vi "xml generate for Q8X.vi"(0 "width1":dbl, 1 "width2":dbl, 2 "single spec":T1={"limit Spec"=array1616x8[12928 elements], "Diff Test Item Name"=["SDD21", "SDD11", "SCD22", "SCC11", "SCD21-SDD21", "NEXT", "ILD_15"], "Spec _Col"=[1, 2, 3, 4, 5, 6, 7]}, 3 "auto get refer point":bool, 4 "input_array_TDD11":string[](array[string]), 5 "input_array_TDD22":string[](array[string]), 6 "input_path_dataSource":path, 7 "input_test_results":bool[](array[boolean]), 8 "show_impspec":string[](array[string]), 10 "路径":path=path "D:/wmgxml.xml", 11 "input_array_time":string[](array[string]), 12 "input_str_label":string, 13 "input_array_impSpec":string[](array[string]), 14 "input_str_CustomerPN":string, 16 "FilePath":string, 17 "FileVer":string, 18 "terminal points":dbl[](array[numeric]), 19 "cable points":dbl[](array[numeric])) -> ()   [LabVIEW 2011]
uses:
  <vilib>/Utility/file.llb/Read From Spreadsheet File (DBL).vi
panel:
  in  "width1 2":dbl
  in  "width2 2":dbl
  in  "cable points 2":dbl[](array[numeric])
  in  "terminal points 4":dbl[](array[numeric])
  in  "auto get refer point 2":bool
  out "terminal points 3":dbl[](array[numeric])
  out "terminal points 2":dbl[](array[numeric])
  out "TestResult":string
  out "TDD":string
  out "NEXT":string
  out "SCC11":string
  out "SCD21-SDD21":string
  out "ILD":string
  out "SDD11":string
  out "SDD21":string
  out "midVar_time":string[](array[string])
  in  "midVar_state":string
  in  "input_str_product":string
  out "midVar_Content":string
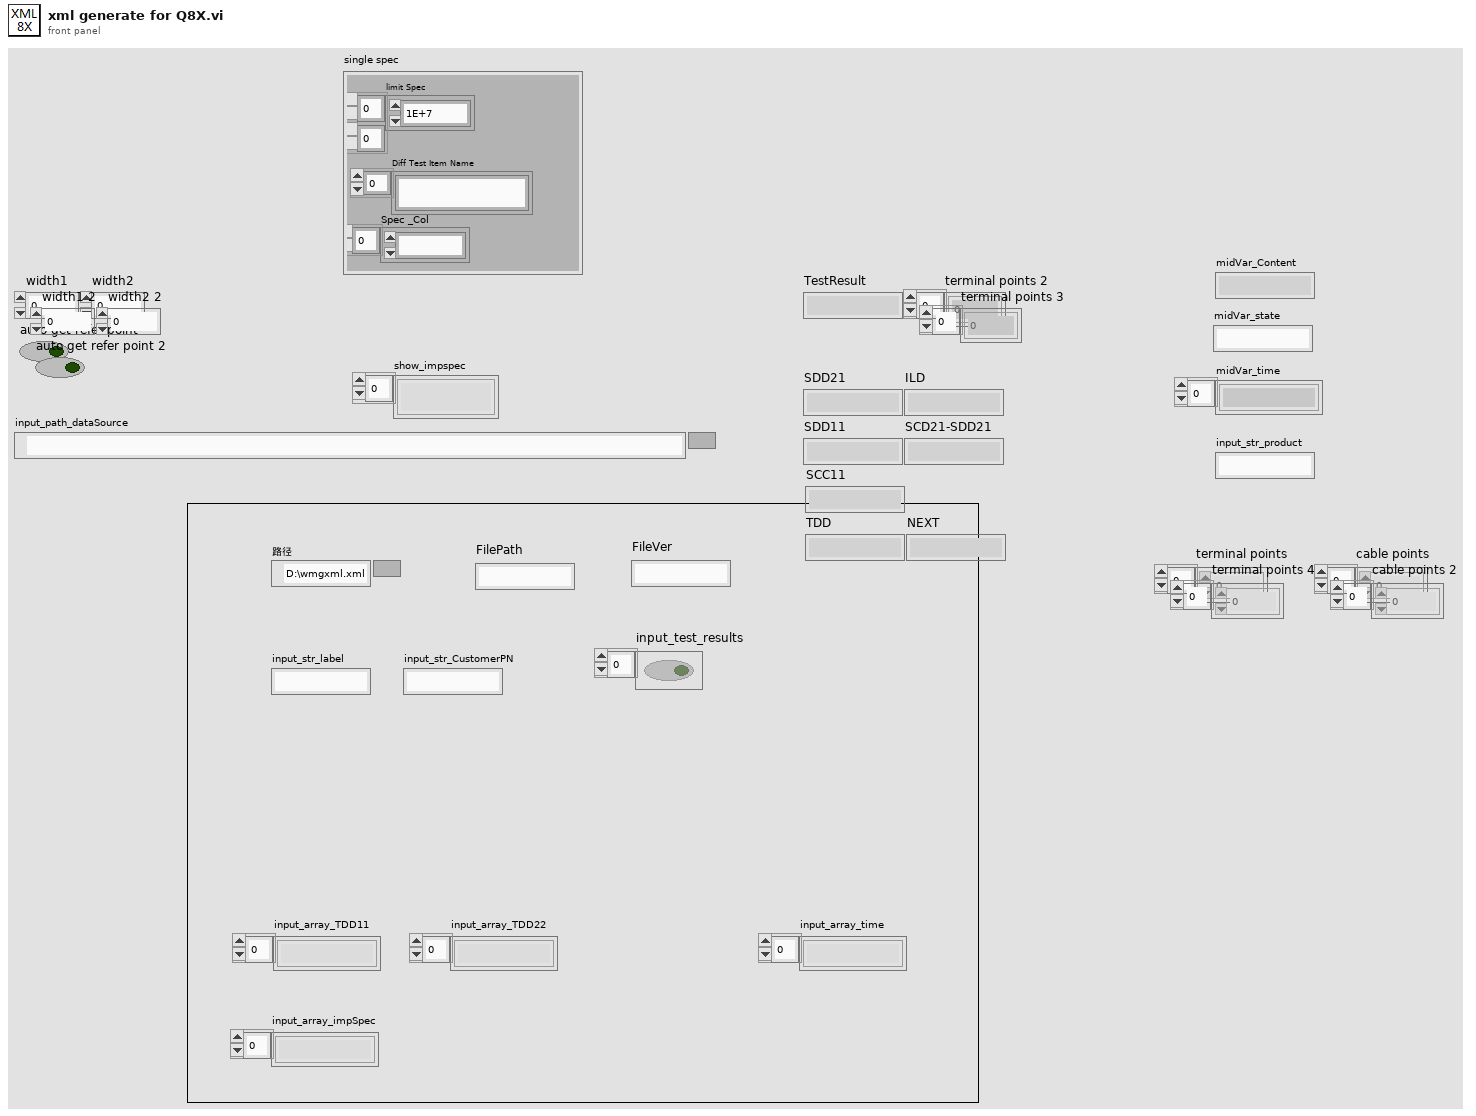
[diagram p1: front panel]
types:
  T1 = cluster{"limit Spec":dbl[][], "Diff Test Item Name":string[], "Spec _Col":i32[]}
  T2 = enum16{"open", "replace", "create", "open or create", "replace or create", "replace or create with confirmation"}
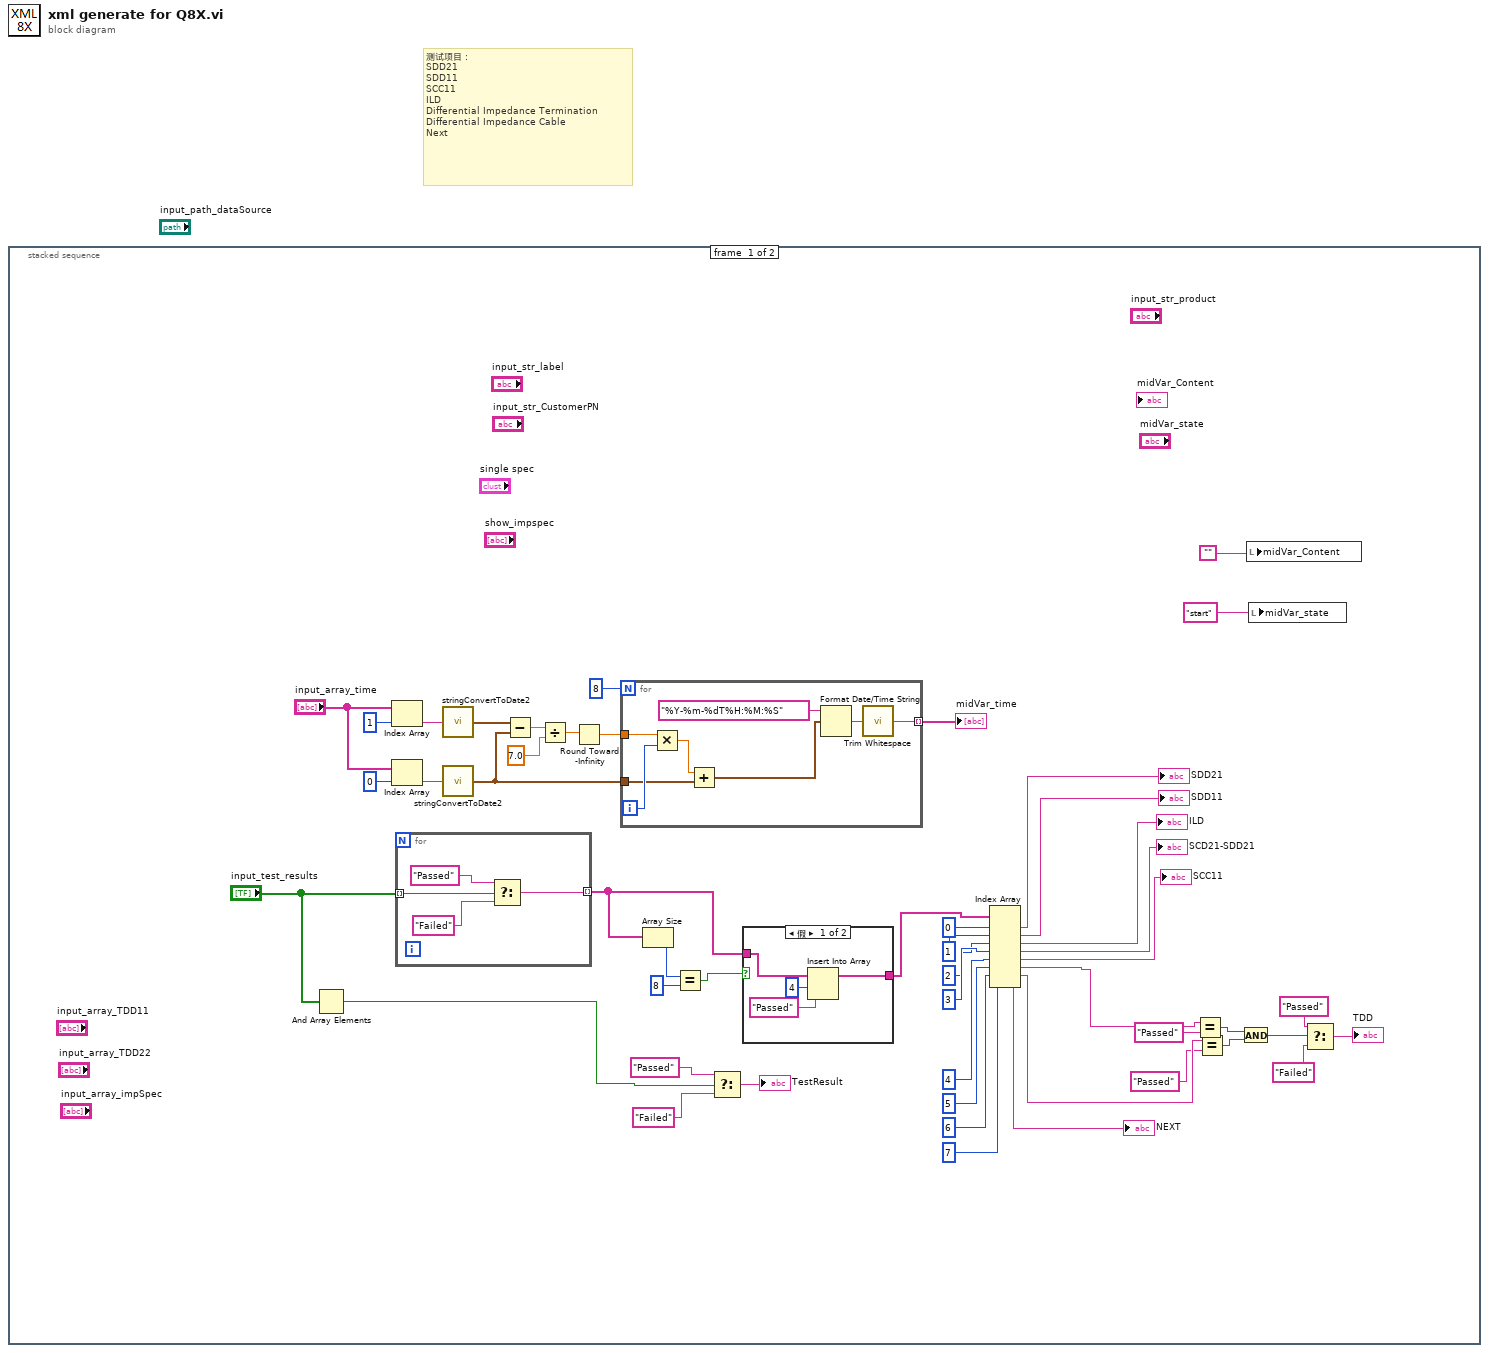
[diagram p0: block diagram]
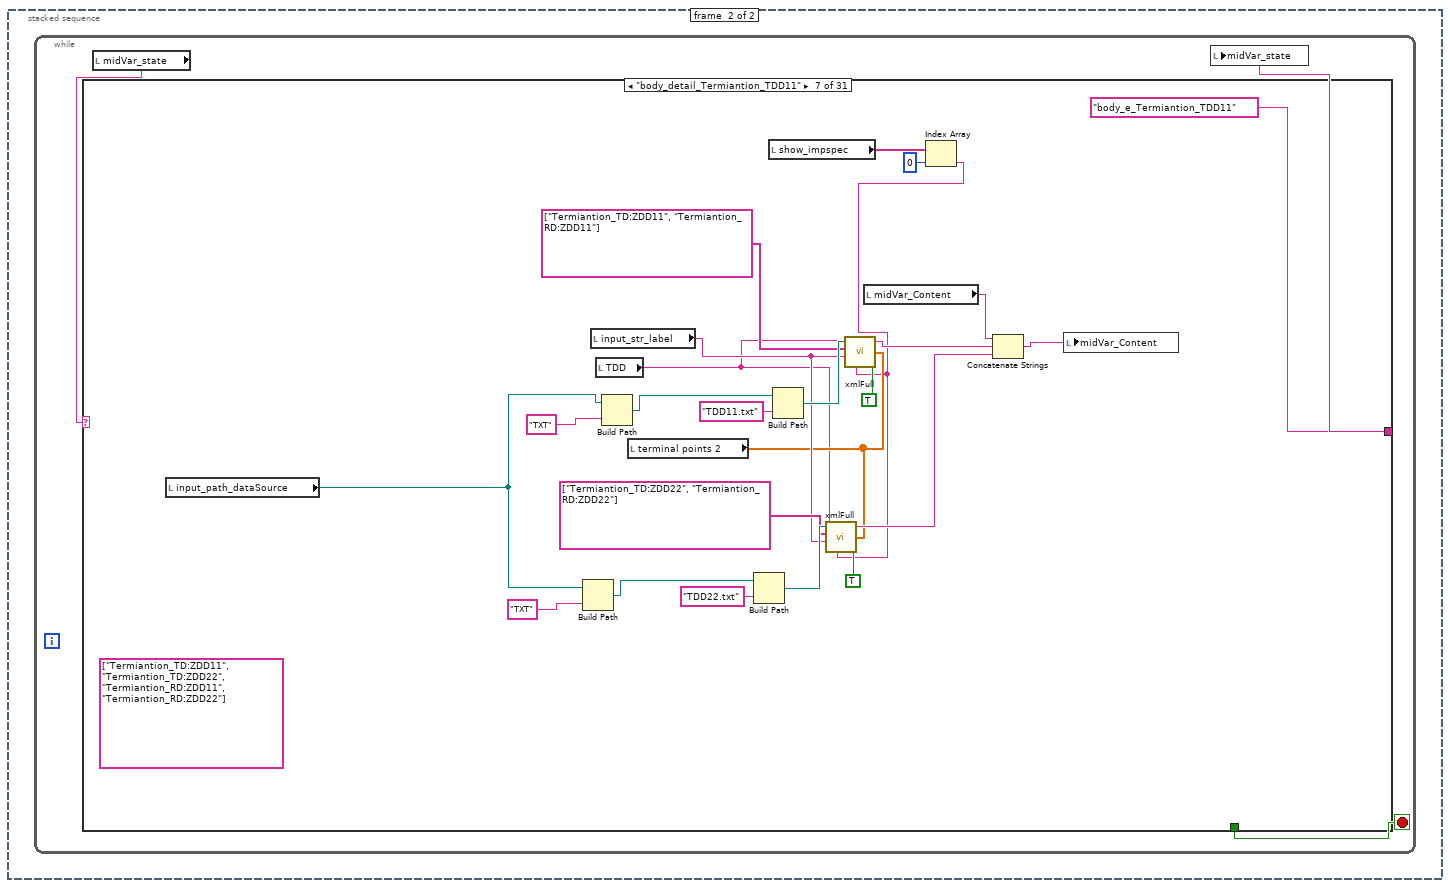
[diagram p3: hidden frame]
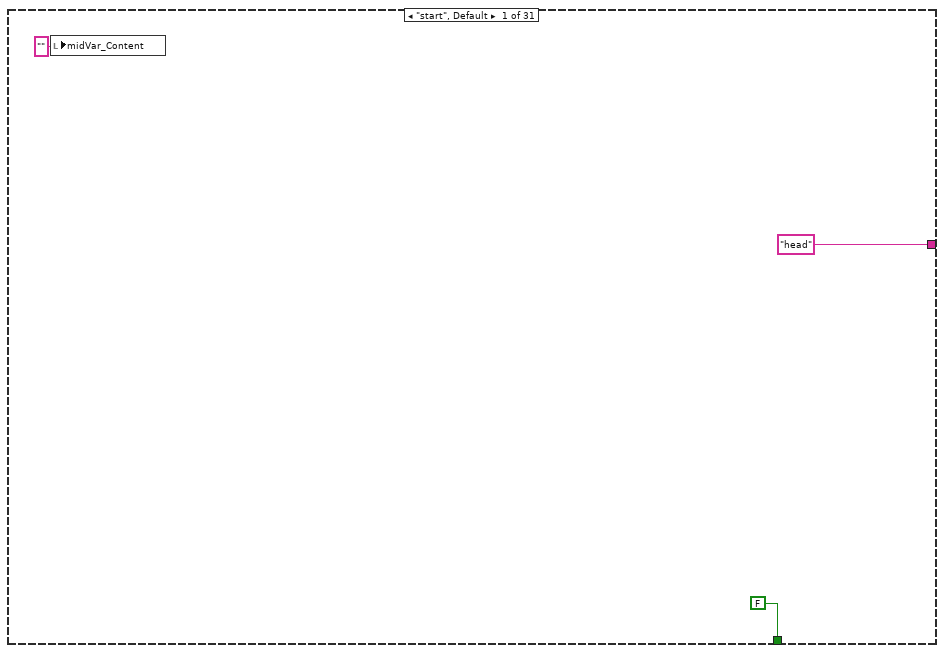
[diagram p4: hidden frame]
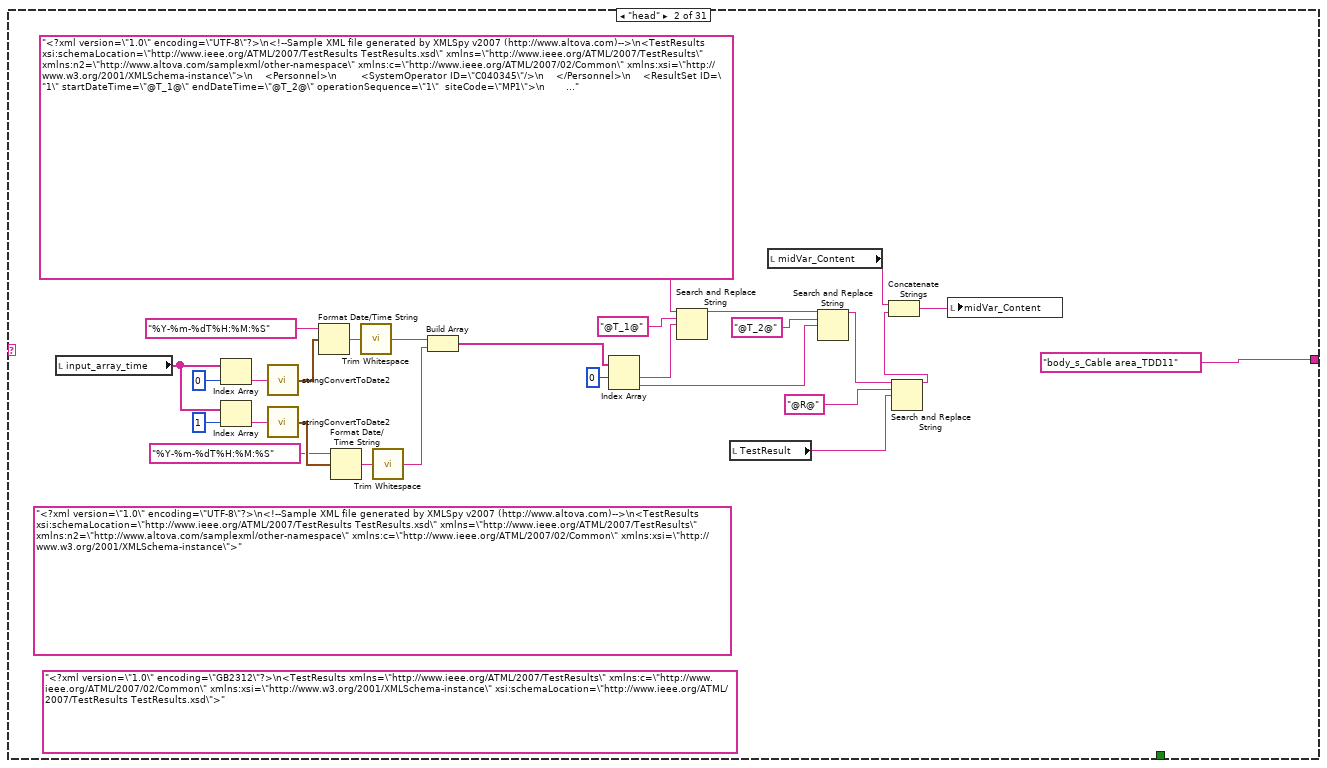
[diagram p5: hidden frame]
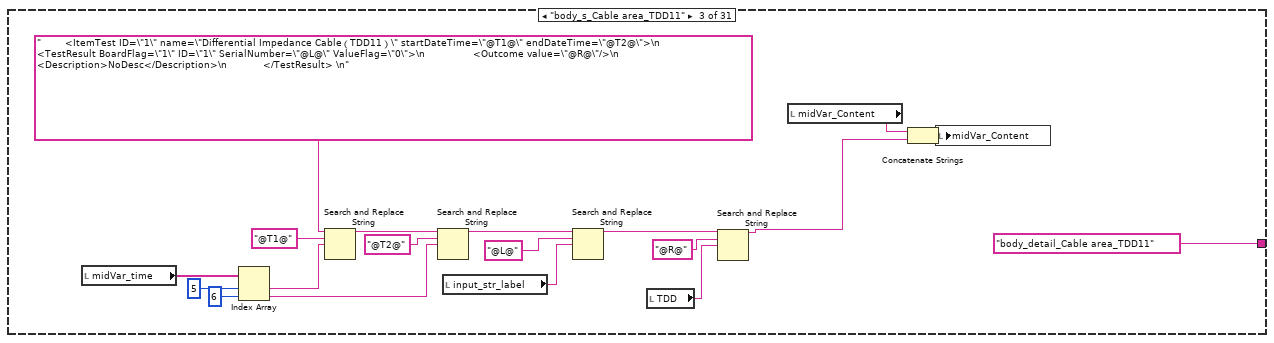
[diagram p6: hidden frame]
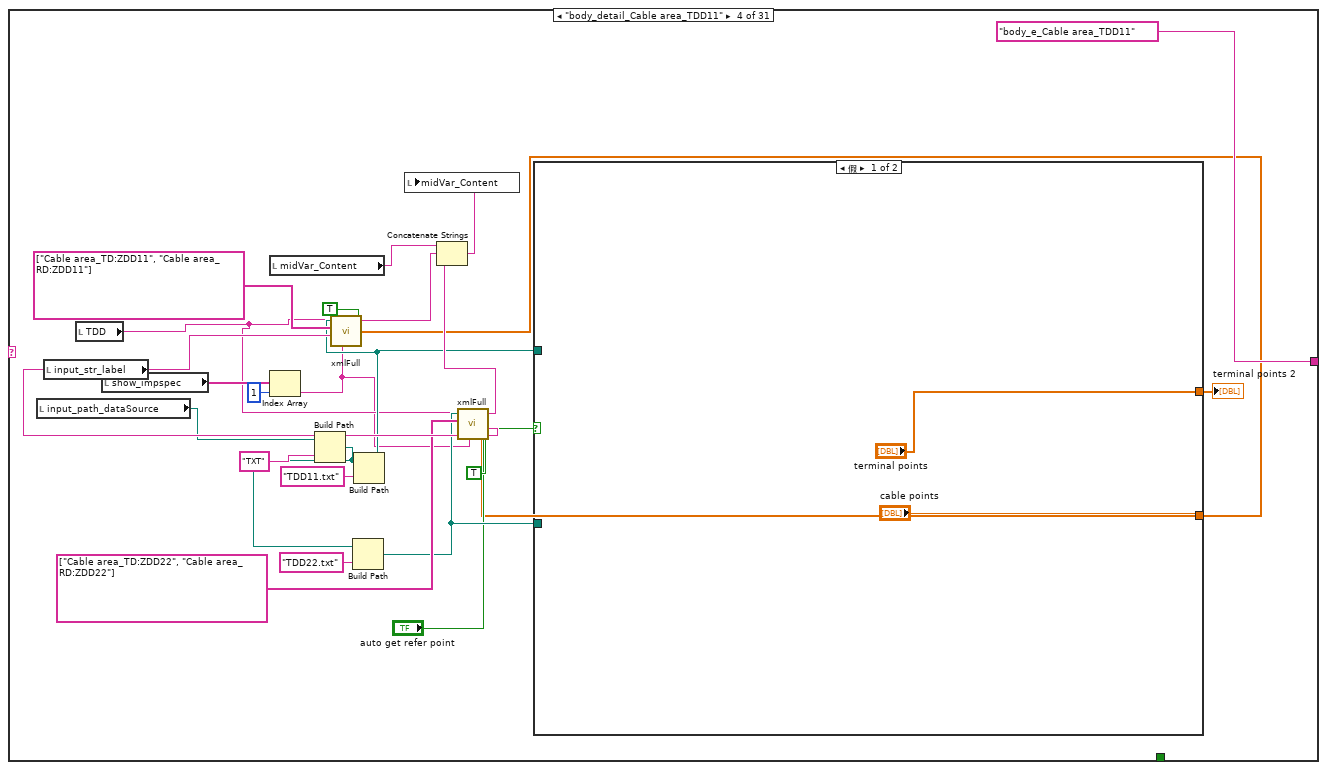
[diagram p7: hidden frame]
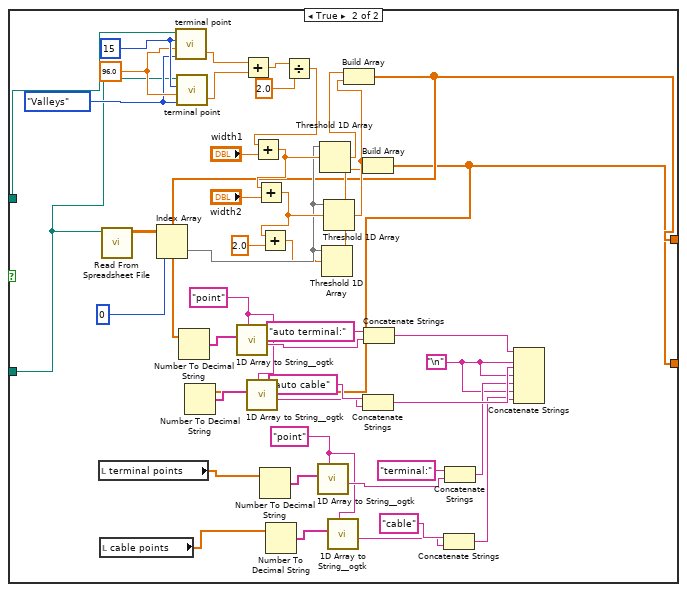
[diagram p8: hidden frame]
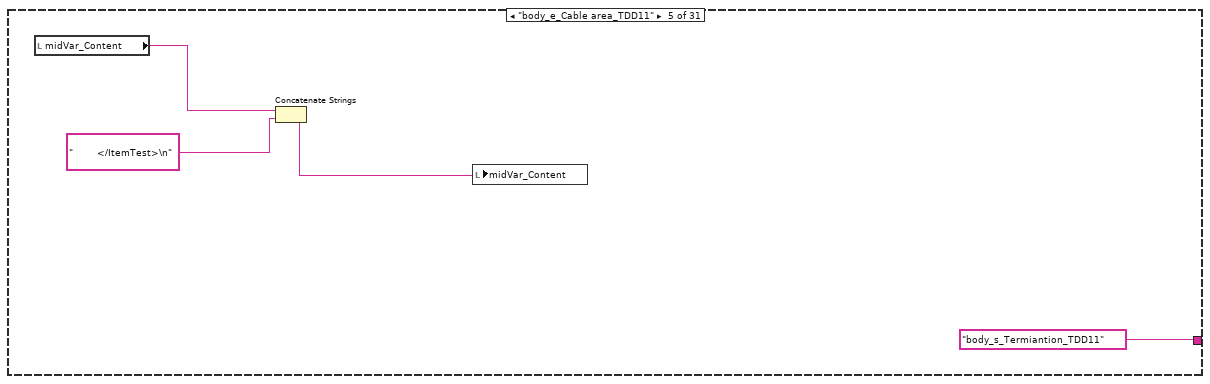
[diagram p9: hidden frame]
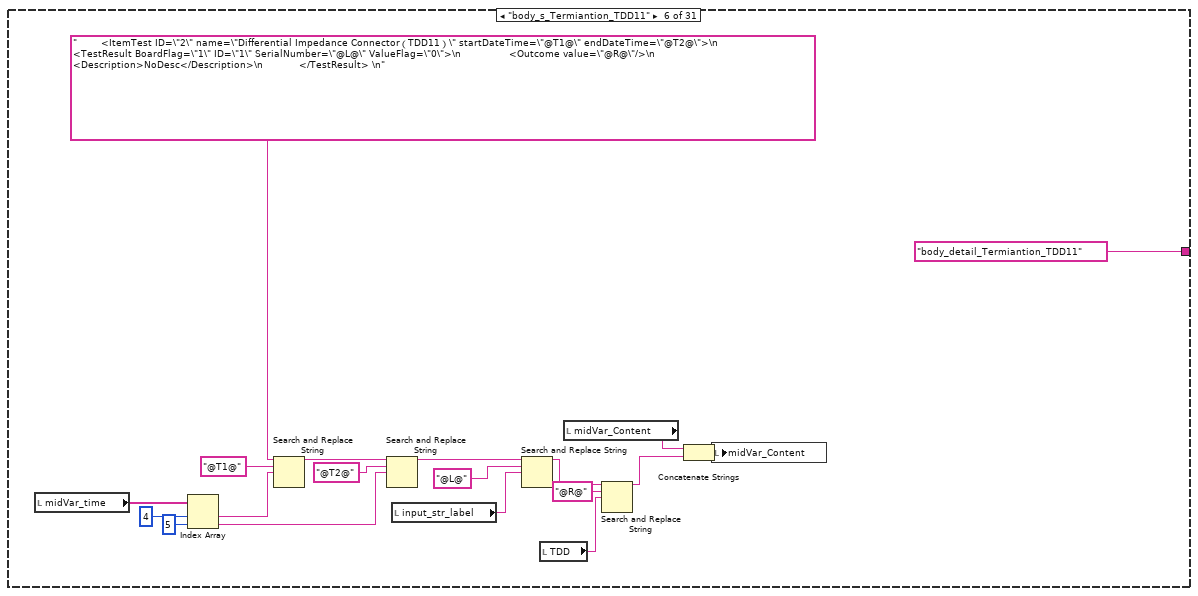
[diagram p10: hidden frame]
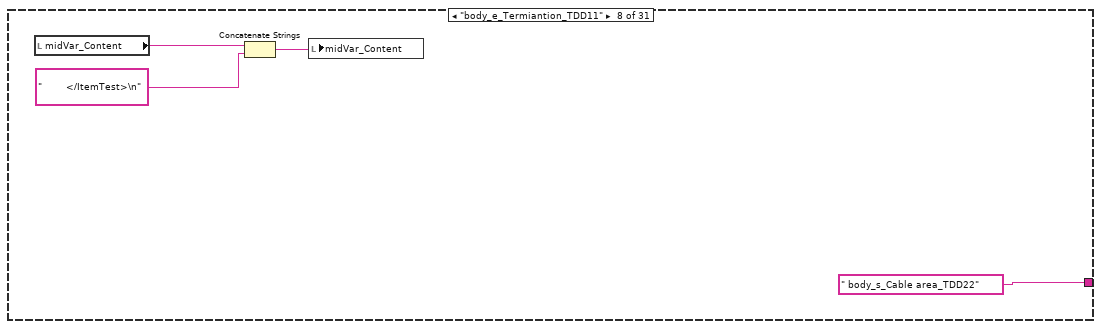
[diagram p11: hidden frame]
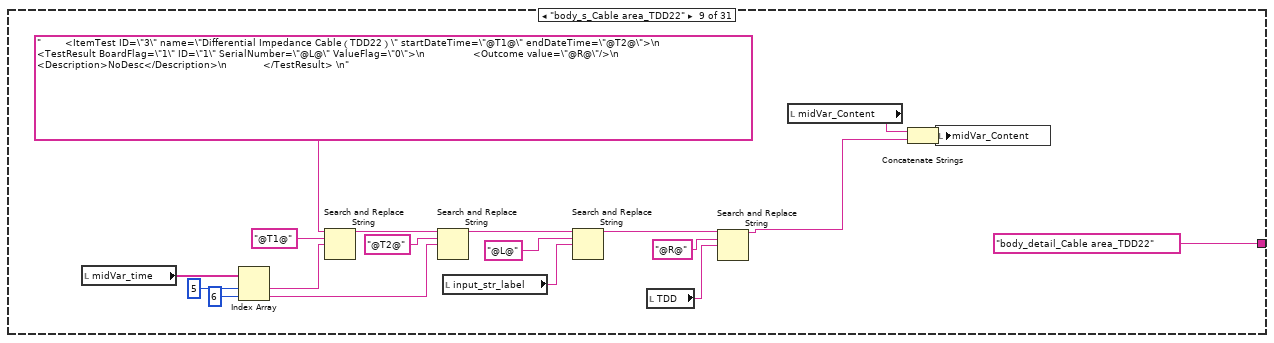
[diagram p12: hidden frame]
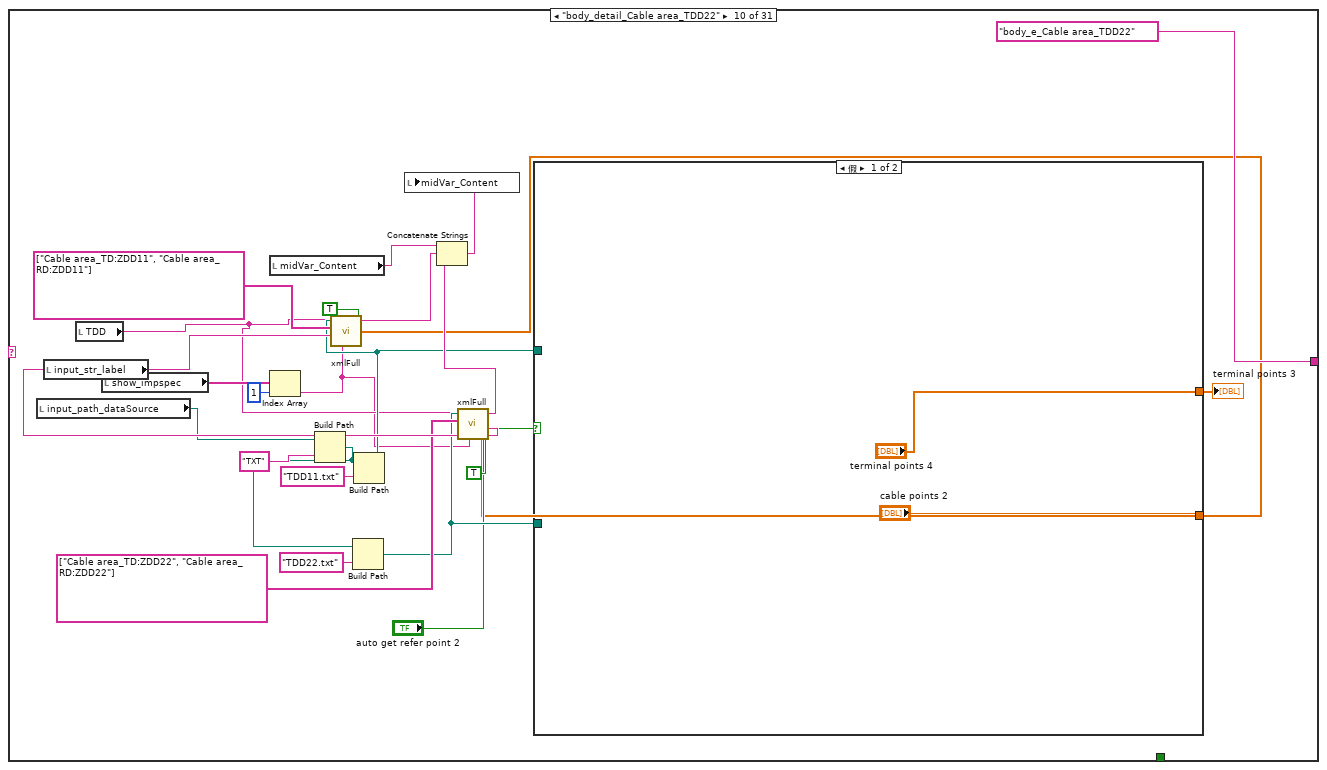
[diagram p13: hidden frame]
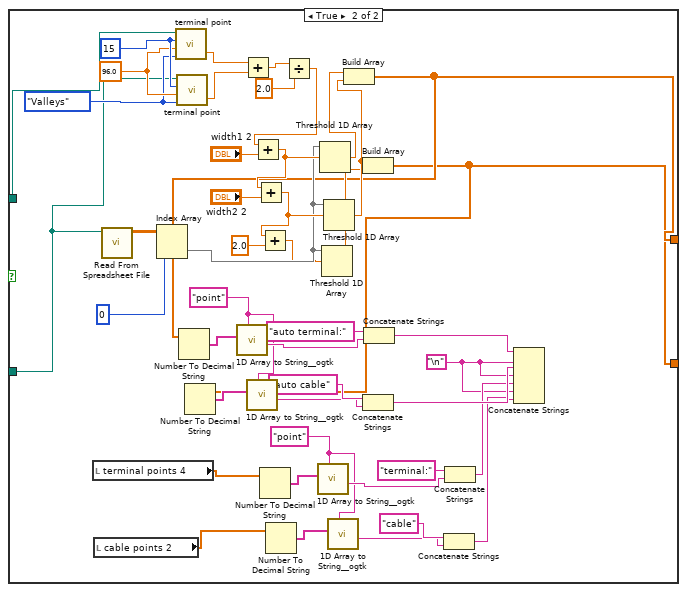
[diagram p14: hidden frame]
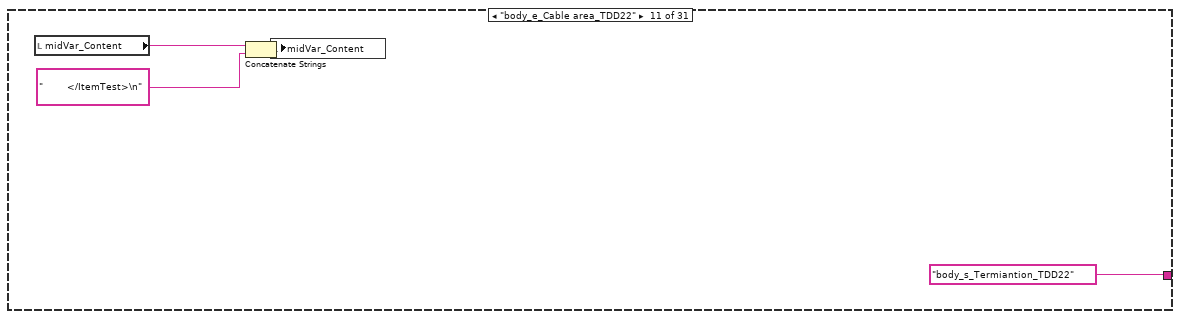
[diagram p15: hidden frame]
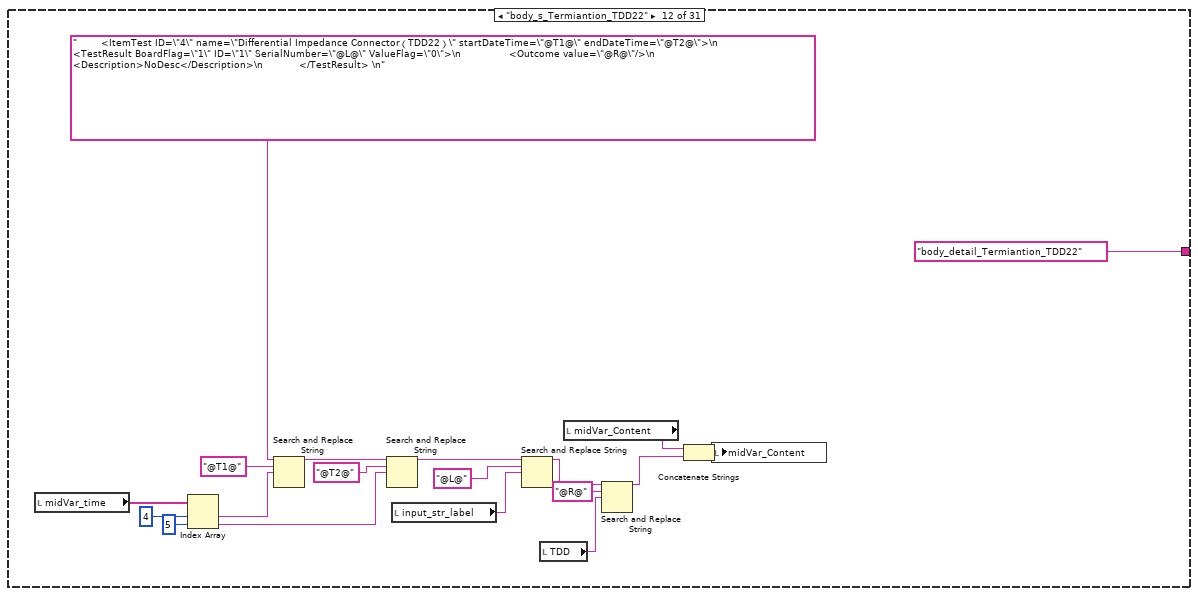
[diagram p16: hidden frame]
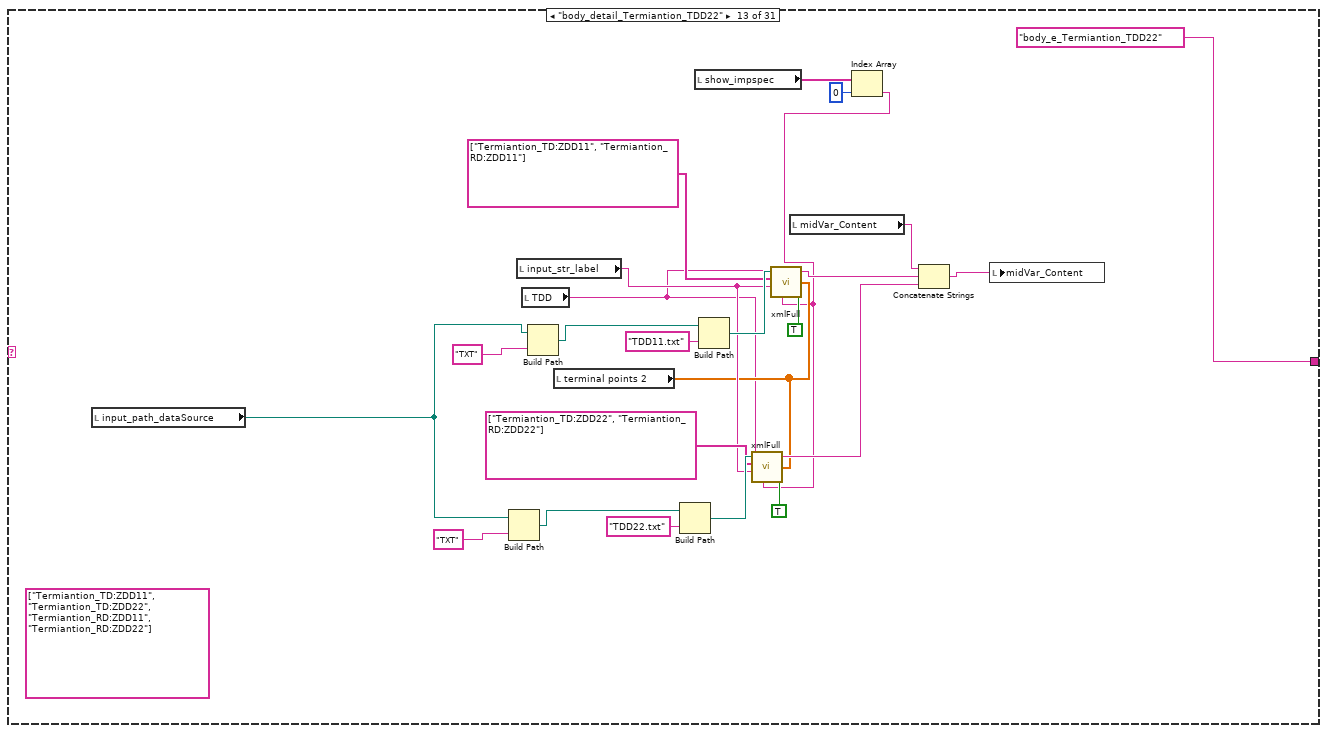
[diagram p17: hidden frame]
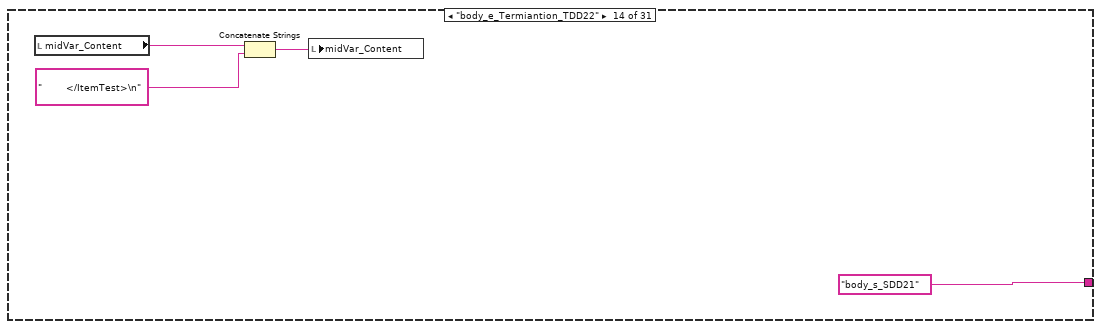
[diagram p18: hidden frame]
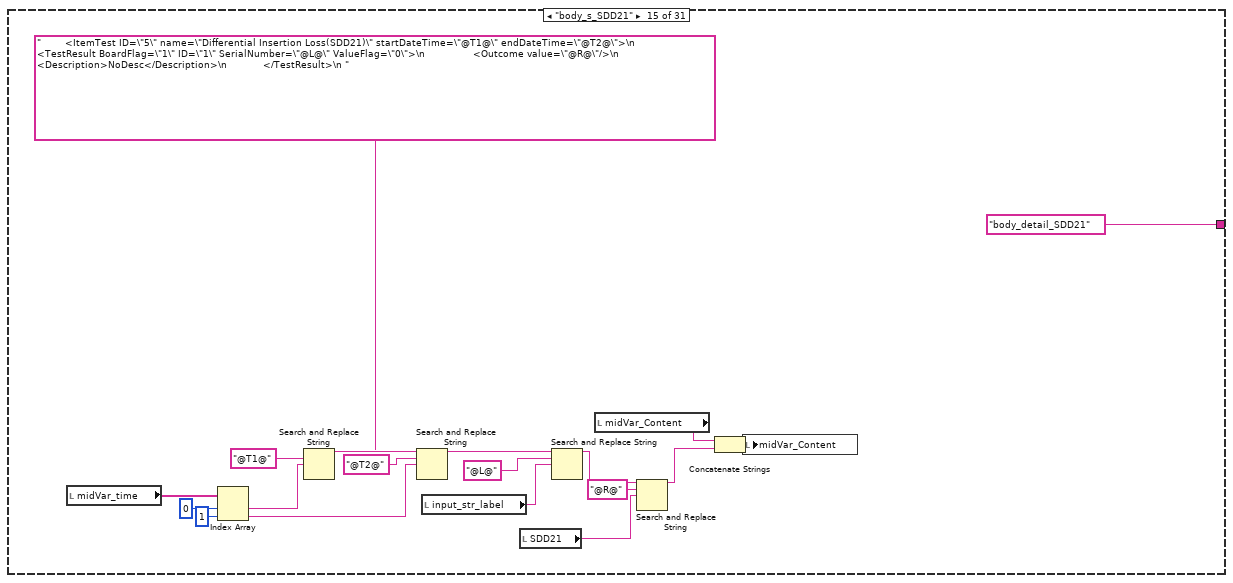
[diagram p19: hidden frame]
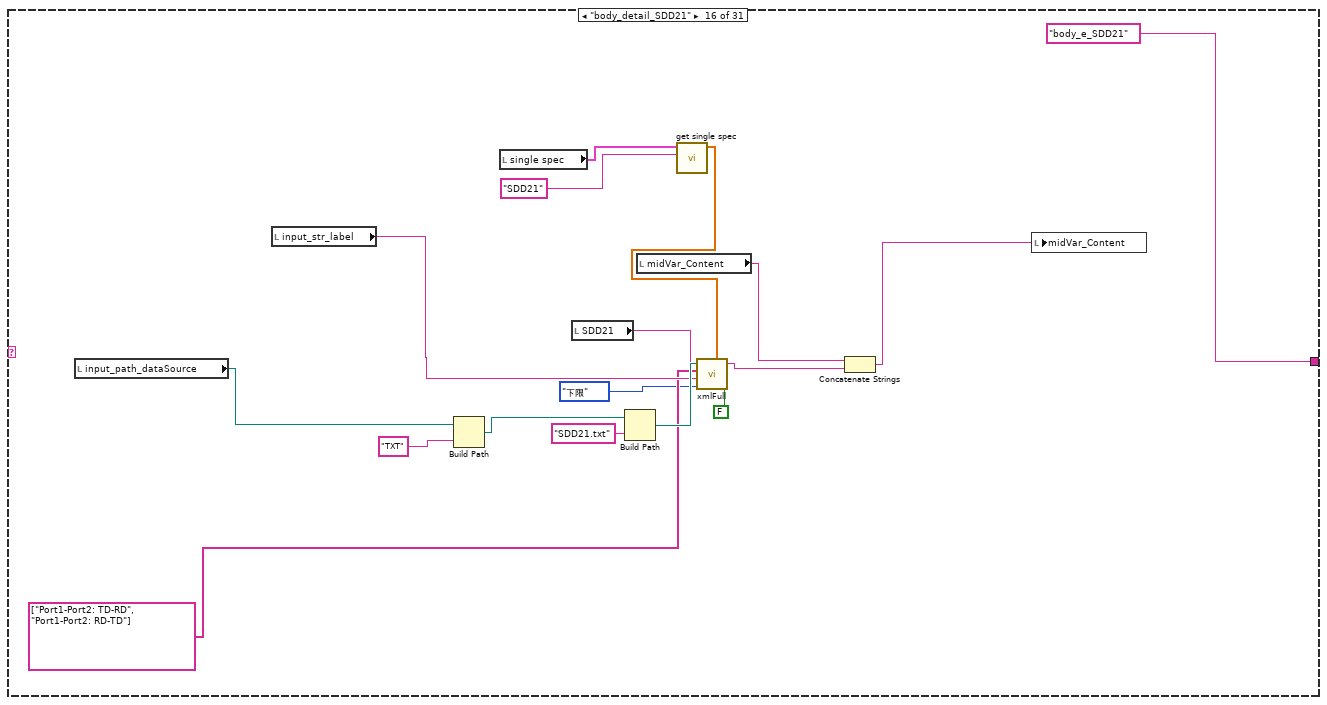
[diagram p20: hidden frame]
diagram:
  # "测试项目：\nSDD21\nSDD11\nSCC11\nILD\nDifferential Impedance Termination\nDifferential Impedance Cable\nNext"
  n1 = stacked-sequence {
    frame #0 {
      n2 = And Array Elements(Boolean array="input_test_results") -> (logical AND=w7:bool)
      n3 = Index Array(array="input_array_time", index=1 ("索引")) -> (element=w38:string)
      n4 = Index Array(array="input_array_time", index=0 ("索引")) -> (element=w39:string)
      n5 = for {
        tunnel: "input_test_results" -> [w58] mode=indexing
        tunnel: [w55] -> w2 mode=indexing
        n6 = Select(t="Passed", s=w58, f="Failed") -> (s? t:f=w55:string)
      }
      n7 = call "stringConvertToDate2.vi"("input_str_yymmdd"=w38) -> ("show_date"=w40:timestamp)
      n8 = call "stringConvertToDate2.vi"("input_str_yymmdd"=w39) -> ("show_date"=w46:timestamp)
      n9 = Subtract(x=w40, y=w46) -> (x-y=w41:dbl)
      n10 = Divide(x=w41, y=7.0) -> (x/y=w43:dbl)
      n11 = Round Toward -Infinity(1:w43) -> (0:w45:dbl)
      n12 = for {
        N: 8 -> [_]
        tunnel: w45 -> [w66]
        tunnel: w46 -> [w64]
        tunnel: [w59] -> w47 mode=indexing
        i -> [w65]
        n13 = Multiply(x=w66, y=w65) -> (x*y=w63:dbl)
        n14 = Add(x=w63, y=w64) -> (x+y=w60:timestamp)
        n15 = Format Date/Time String(time format string (%c)="%Y-%m-%dT%H:%M:%S" ("时间格式字符串(%c)"), seconds (now)=w60) -> (date/time string=w61:string)  [unwired: 1 in]
        n16 = call <vilib>:"Trim Whitespace.vi"("string"=w61) -> ("trimmed string"=w59:string)  [unwired: 1 in]
      }
      "midVar_time" <- w47
      n17 = Array Size(array=w2) -> (size(s)=w5:i32)
      n18 = Equal?(x=w5, y=8) -> (x = y?=w3:bool)
      n19 = Select(t="Passed", s=w7, f="Failed") -> (s? t:f=→"TestResult":string)
      n20 = case shown="假" w3 {
        tunnel: w2 -> [w53 w54]
        tunnel: [w50 w54] -> w1
        frame False {
          n21 = Insert Into Array(array=w53, index=4 ("索引"), new element="Passed" ("新元素/子数组")) -> (w50:string[])
        }
        frame True {
        }
      }
      n22 = Index Array(array=w1, index #1=0 ("索引"), index #2=1 ("索引"), index #3=2 ("索引"), index #4=3 ("索引"), index #5=4 ("索引"), index #6=5 ("索引"), index #7=6 ("索引"), index #8=7 ("索引")) -> (element #1=→"SDD21":string, element #2=→"SDD11":string, element #3=→"ILD":string, element #4=→"SCD21-SDD21":string, element #5=→"SCC11":string, element #6=w20:string, element #7=w18:string, element #8=→"NEXT":string)
      n23 = Equal?(x=w20, y="Passed") -> (x = y?=w16:bool)
      n24 = Equal?(x=w18, y="Passed") -> (x = y?=w15:bool)
      n25 = And(x=w16, y=w15) -> (x .and. y?=w14:bool)
      n26 = local write "midVar_Content"("") -> ()
      n27 = local write "midVar_state"("start" ("state")) -> ()
      n28 = Select(t="Passed", s=w14, f="Failed") -> (s? t:f=→"TDD":string)
    }
    frame #1 {
      n29 = while {
        stop <- w67 stop-if-true
        n30 = local read "midVar_state"() -> (w69:string)
        n31 = case shown="\"body_detail_Termiantion_TDD11\"" w69 {
          tunnel: ["head" ("state") "body_s_Cable area_TDD11" ("state") "body_detail_Cable area_TDD11" "body_e_Cable area_TDD11" "body_s_Termiantion_TDD11" "body_detail_Termiantion_TDD11" "body_e_Termiantion_TDD11" " body_s_Cable area_TDD22" "body_detail_Cable area_TDD22" "body_e_Cable area_TDD22" "body_s_Termiantion_TDD22" "body_detail_Termiantion_TDD22" "body_e_Termiantion_TDD22" "body_s_SDD21" "body_detail_SDD21" "body_e_SDD21" "body_s_SDD11" "body_detail_SDD11" "body_e_SDD11" "body_s_Next" "body_detail_Next" "body_e_Next" "body_s_SCD21" "body_detail_SCD21" "body_e_SCD21" "body_s_SCD21-SDD21" "body_detail_SCD21-SDD21" "body_e_SCD21-SDD21" "tail" "end" ("state") "start" ("state")] -> w68
          tunnel: [FALSE _ _ _ _ _ _ _ _ _ _ _ _ _ _ _ _ _ _ _ _ _ _ _ _ _ _ _ _ _ TRUE] -> w67
          frame "start", Default {
            n32 = local write "midVar_Content"("" ("字符串")) -> ()
          }
          frame "head" {
            (unwired) "<?xml version=\"1.0\" encoding=\"GB2312\"?>\n<TestResults xmlns=\"http://www.ieee.org/ATML/2007/TestResults\" xmlns:c=\"http://www.ieee.org/ATML/2007/02/Common\" xmlns:xsi=\"http://www.w3.org/2001/XMLSchema-instance\" xsi:schemaLocation=\"http://www.ieee.org/ATML/2007/TestResults TestResults.xsd\">"
            (unwired) "<?xml version=\"1.0\" encoding=\"UTF-8\"?>\n<!--Sample XML file generated by XMLSpy v2007 (http://www.altova.com)-->\n<TestResults xsi:schemaLocation=\"http://www.ieee.org/ATML/2007/TestResults TestResults.xsd\" xmlns=\"http://www.ieee.org/ATML/2007/TestResults\" xmlns:n2=\"http://www.altova.com/samplexml/other-namespace\" xmlns:c=\"http://www.ieee.org/ATML/2007/02/Common\" xmlns:xsi=\"http://www.w3.org/2001/XMLSchema-instance\">"
            n33 = local read "input_array_time"() -> (w86:string[])
            n34 = Index Array(array=w86, index=0 ("索引")) -> (element=w85:string)
            n35 = Index Array(array=w86, index=1 ("索引")) -> (element=w84:string)
            n36 = call "stringConvertToDate2.vi"("input_str_yymmdd"=w85) -> ("show_date"=w82:timestamp)
            n37 = call "stringConvertToDate2.vi"("input_str_yymmdd"=w84) -> ("show_date"=w81:timestamp)
            n38 = Format Date/Time String(time format string (%c)="%Y-%m-%dT%H:%M:%S" ("时间格式字符串(%c)"), seconds (now)=w82) -> (date/time string=w89:string)  [unwired: 1 in]
            n39 = Format Date/Time String(time format string (%c)="%Y-%m-%dT%H:%M:%S" ("时间格式字符串(%c)"), seconds (now)=w81) -> (date/time string=w83:string)  [unwired: 1 in]
            n40 = call <vilib>:"Trim Whitespace.vi"("string"=w89) -> ("trimmed string"=w79:string)  [unwired: 1 in]
            n41 = call <vilib>:"Trim Whitespace.vi"("string"=w83) -> ("trimmed string"=w78:string)  [unwired: 1 in]
            n42 = Build Array(w79, w78) -> (w77:string[])
            n43 = Index Array(array=w77, index #1=0 ("索引")) -> (element #1=w98:string, element #2=w95:string)  [unwired: 1 in]
            n44 = Search and Replace String(input string="<?xml version=\"1.0\" encoding=\"UTF-8\"?>\n<!--Sample XML file generated by XMLSpy v2007 (http://www.altova.com)-->\n<TestResults xsi:schemaLocation=\"http://www.ieee.org/ATML/2007/TestResults TestResults.xsd\" xmlns=\"http://www.ieee.org/ATML/2007/TestResults\" xmlns:n2=\"http://www.altova.com/samplexml/other-namespace\" xmlns:c=\"http://www.ieee.org/ATML/2007/02/Common\" xmlns:xsi=\"http://www.w3.org/2001/XMLSchema-instance\">\n    <Personnel>\n        <SystemOperator ID=\"C040345\"/>\n    </Personnel>\n    <ResultSet ID=\"1\" startDateTime=\"@T_1@\" endDateTime=\"@T_2@\" operationSequence=\"1\"  siteCode=\"MP1\">\n        <Description>CMZ00A2R</Description>\n        <TestResult BoardFlag=\"1\" ID=\"1\">\n            <Outcome value=\"@R@\"/>\n        </TestResult>\n", search string="@T_1@" ("搜索字符串"), replace string=w98) -> (result string=w97:string)  [unwired: 5 in, 3 out]
            n45 = local read "TestResult"() -> (w73:string)
            n46 = local read "midVar_Content"() -> (w93:string)
            n47 = Search and Replace String(input string=w97, search string="@T_2@" ("搜索字符串"), replace string=w95) -> (result string=w76:string)  [unwired: 5 in, 3 out]
            n48 = Search and Replace String(input string=w76, search string="@R@" ("搜索字符串"), replace string=w73) -> (result string=w75:string)  [unwired: 5 in, 3 out]
            n49 = Concatenate Strings(w93, w75) -> (w92:string)
            n50 = local write "midVar_Content"(w92) -> ()
          }
          frame "body_s_Cable area_TDD11" {
            n51 = local read "midVar_time"() -> (w106:string[])
            n52 = Index Array(array=w106, index #1=5 ("索引"), index #2=6 ("索引")) -> (element #1=w117:string, element #2=w114:string)
            n53 = Search and Replace String(input string="        <ItemTest ID=\"1\" name=\"Differential Impedance Cable（TDD11）\" startDateTime=\"@T1@\" endDateTime=\"@T2@\">\n            <TestResult BoardFlag=\"1\" ID=\"1\" SerialNumber=\"@L@\" ValueFlag=\"0\">\n                <Outcome value=\"@R@\"/>\n                <Description>NoDesc</Description>\n            </TestResult> \n", search string="@T1@" ("搜索字符串"), replace string=w117) -> (result string=w116:string)  [unwired: 5 in, 3 out]
            n54 = Search and Replace String(input string=w116, search string="@T2@" ("搜索字符串"), replace string=w114) -> (result string=w109:string)  [unwired: 5 in, 3 out]
            n55 = local read "input_str_label"() -> (w108:string)
            n56 = Search and Replace String(input string=w109, search string="@L@" ("搜索字符串"), replace string=w108) -> (result string=w104:string)  [unwired: 5 in, 3 out]
            n57 = local read "TDD"() -> (w101:string)
            n58 = Search and Replace String(input string=w104, search string="@R@" ("搜索字符串"), replace string=w101) -> (result string=w103:string)  [unwired: 5 in, 3 out]
            n59 = local read "midVar_Content"() -> (w113:string)
            n60 = Concatenate Strings(w113, w103) -> (w112:string)
            n61 = local write "midVar_Content"(w112) -> ()
          }
          frame "body_detail_Cable area_TDD11" {
            n62 = local read "input_path_dataSource"() -> (w132:path)
            n63 = local read "input_str_label"() -> (w135:string)
            n64 = local read "TDD"() -> (w121:string)
            n65 = local read "show_impspec"() -> (w123:string[])
            n66 = local read "midVar_Content"() -> (w142:string)
            n67 = Index Array(array=w123, index=1 ("索引")) -> (element=w120:string)
            n68 = Build Path(base path=w132, name or relative path="TXT" ("名称或相对路径")) -> (appended path=w131:path)
            n69 = Build Path(base path=w131, name or relative path="TDD22.txt" ("名称或相对路径")) -> (appended path=w128:path)
            n70 = Build Path(base path=w131, name or relative path="TDD11.txt" ("名称或相对路径")) -> (appended path=w127:path)
            n71 = case shown="假" "auto get refer point" {
              tunnel: w128 -> [_ w178]
              tunnel: w127 -> [_ w190]
              tunnel: ["cable points" w151] -> w124
              tunnel: ["terminal points" w152] -> w125
              frame False {
              }
              frame True {
                w147 = "\n"
                w155 = "point" ("delimiter (Tab)")
                w164 = "point" ("delimiter (Tab)")
                w187 = enum32{"Peaks", "Valleys"}."Valleys" ("peaks/valleys")
                w188 = 96.0 ("threshold")
                w189 = 15 ("PD width")
                n72 = local read "terminal points"() -> (w160:dbl[])
                n73 = local read "cable points"() -> (w161:dbl[])
                n74 = call-poly <vilib>:"Read From Spreadsheet File.vi"("file path (dialog if empty)"=w178) -> ("all rows"=w177:dbl[][])  [unwired: 6 in, 4 out]
                n75 = Index Array(array=w177, index (col)=0 ("禁用的索引 (列)")) -> (element=w173:dbl[])  [unwired: 1 in]
                n76 = call "terminal point.vi"("peaks/valleys"=w187, "threshold"=w188, "PD width"=w189, "TDD filePath"=w190) -> ("time low"=w182:dbl)  [unwired: 1 out]
                n77 = call "terminal point.vi"("peaks/valleys"=w187, "threshold"=w188, "PD width"=w189, "TDD filePath"=w178) -> ("time low"=w181:dbl)  [unwired: 1 out]
                n78 = Add(x=w182, y=w181) -> (x+y=w186:dbl)
                n79 = Number To Decimal String(number=w160) -> (decimal integer string=w162:string[])  [unwired: 1 in]
                n80 = Number To Decimal String(number=w161) -> (decimal integer string=w163:string[])  [unwired: 1 in]
                n81 = Divide(x=w186, y=2.0) -> (x/y=w179:dbl)
                n82 = Add(x=w179, y="width1") -> (x+y=w175:dbl)
                n83 = Add(x=w175, y="width2") -> (x+y=w174:dbl)
                n84 = Add(x=w174, y=2.0) -> (x+y=w172:dbl)
                n85 = call <userlib>:"1D Array to String__ogtk.vi"("delimiter (Tab)"=w164, "Array of Strings"=w162) -> ("delimited string"=w166:string)  [unwired: 9 in]
                n86 = Threshold 1D Array(2:w175, 3:w173) -> (0:w171:dbl)  [unwired: 1 in]
                n87 = Threshold 1D Array(2:w172, 3:w173) -> (0:w169:dbl)  [unwired: 1 in]
                n88 = Threshold 1D Array(2:w174, 3:w173) -> (0:w170:dbl)  [unwired: 1 in]
                n89 = call <userlib>:"1D Array to String__ogtk.vi"("delimiter (Tab)"=w164, "Array of Strings"=w163) -> ("delimited string"=w167:string)  [unwired: 9 in]
                n90 = Build Array(w171, w170) -> (w152:dbl[])
                n91 = Number To Decimal String(number=w152) -> (decimal integer string=w153:string[])  [unwired: 1 in]
                n92 = call <userlib>:"1D Array to String__ogtk.vi"("delimiter (Tab)"=w155, "Array of Strings"=w153) -> ("delimited string"=w157:string)  [unwired: 9 in]
                n93 = Build Array(w170, w169) -> (w151:dbl[])
                n94 = Number To Decimal String(number=w151) -> (decimal integer string=w154:string[])  [unwired: 1 in]
                n95 = call <userlib>:"1D Array to String__ogtk.vi"("delimiter (Tab)"=w155, "Array of Strings"=w154) -> ("delimited string"=w158:string)  [unwired: 9 in]
                n96 = Concatenate Strings("auto cable" ("字符串"), w158) -> (w149:string)
                n97 = Concatenate Strings("auto terminal:" ("字符串"), w157) -> (w150:string)
                n98 = Concatenate Strings("cable" ("字符串"), w167) -> (w146:string)
                n99 = Concatenate Strings("terminal:" ("字符串"), w166) -> (w148:string)
                n100 = Concatenate Strings(w150, w147, w149, w147, w148, w147, w146) -> ()  [unwired: 1 out]
              }
            }
            "terminal points 2" <- w125
            n101 = call "xmlFull.vi"("TDD?"=TRUE, "Points"=w124, "file path (dialog if empty)"=w127, "TDD spec"=w120, "SN"=w135, "数组"=string[] ["Cable area_TD:ZDD11", "Cable area_RD:ZDD11"], "second result"=w121) -> ("OutPutXml"=w140:string)  [unwired: 3 in]
            n102 = call "xmlFull.vi"("TDD?"=TRUE, "Points"=w124, "file path (dialog if empty)"=w128, "TDD spec"=w120, "SN"=w135, "数组"=string[] ["Cable area_TD:ZDD22", "Cable area_RD:ZDD22"], "second result"=w121) -> ("OutPutXml"=w133:string)  [unwired: 3 in]
            n103 = Concatenate Strings(w142, w140, w133) -> (w141:string)
            n104 = local write "midVar_Content"(w141) -> ()
          }
          frame "body_e_Cable area_TDD11" {
            n105 = local read "midVar_Content"() -> (w194:string)
            n106 = Concatenate Strings(w194, "        </ItemTest>\n") -> (w193:string)
            n107 = local write "midVar_Content"(w193) -> ()
          }
          frame "body_s_Termiantion_TDD11" {
            n108 = local read "midVar_time"() -> (w200:string[])
            n109 = Index Array(array=w200, index #1=4 ("索引"), index #2=5 ("索引")) -> (element #1=w211:string, element #2=w208:string)
            n110 = Search and Replace String(input string="        <ItemTest ID=\"2\" name=\"Differential Impedance Connector（TDD11）\" startDateTime=\"@T1@\" endDateTime=\"@T2@\">\n            <TestResult BoardFlag=\"1\" ID=\"1\" SerialNumber=\"@L@\" ValueFlag=\"0\">\n                <Outcome value=\"@R@\"/>\n                <Description>NoDesc</Description>\n            </TestResult> \n", search string="@T1@" ("搜索字符串"), replace string=w211) -> (result string=w210:string)  [unwired: 5 in, 3 out]
            n111 = Search and Replace String(input string=w210, search string="@T2@" ("搜索字符串"), replace string=w208) -> (result string=w203:string)  [unwired: 5 in, 3 out]
            n112 = local read "input_str_label"() -> (w202:string)
            n113 = Search and Replace String(input string=w203, search string="@L@" ("搜索字符串"), replace string=w202) -> (result string=w198:string)  [unwired: 5 in, 3 out]
            n114 = local read "TDD"() -> (w195:string)
            n115 = local read "midVar_Content"() -> (w207:string)
            n116 = Search and Replace String(input string=w198, search string="@R@" ("搜索字符串"), replace string=w195) -> (result string=w197:string)  [unwired: 5 in, 3 out]
            n117 = Concatenate Strings(w207, w197) -> (w206:string)
            n118 = local write "midVar_Content"(w206) -> ()
          }
          frame "body_detail_Termiantion_TDD11" {
            (unwired) string[] ["Termiantion_TD:ZDD11", "Termiantion_TD:ZDD22", "Termiantion_RD:ZDD11", "Termiantion_RD:ZDD22"]
            n119 = local read "input_path_dataSource"() -> (w224:path)
            n120 = Build Path(base path=w224, name or relative path="TXT" ("名称或相对路径")) -> (appended path=w231:path)
            n121 = local read "input_str_label"() -> (w221:string)
            n122 = local read "TDD"() -> (w217:string)
            n123 = Build Path(base path=w224, name or relative path="TXT" ("名称或相对路径")) -> (appended path=w235:path)
            n124 = local read "terminal points 2"() -> (w218:dbl[])
            n125 = Build Path(base path=w231, name or relative path="TDD22.txt" ("名称或相对路径")) -> (appended path=w229:path)
            n126 = local read "show_impspec"() -> (w216:string[])
            n127 = Build Path(base path=w235, name or relative path="TDD11.txt" ("名称或相对路径")) -> (appended path=w233:path)
            n128 = local read "midVar_Content"() -> (w219:string)
            n129 = Index Array(array=w216, index=0 ("索引")) -> (element=w214:string)
            n130 = call "xmlFull.vi"("TDD?"=TRUE, "Points"=w218, "file path (dialog if empty)"=w229, "TDD spec"=w214, "SN"=w221, "数组"=string[] ["Termiantion_TD:ZDD22", "Termiantion_RD:ZDD22"], "second result"=w217) -> ("OutPutXml"=w227:string)  [unwired: 3 in]
            n131 = call "xmlFull.vi"("TDD?"=TRUE, "Points"=w218, "file path (dialog if empty)"=w233, "TDD spec"=w214, "SN"=w221, "数组"=string[] ["Termiantion_TD:ZDD11", "Termiantion_RD:ZDD11"], "second result"=w217) -> ("OutPutXml"=w228:string)  [unwired: 3 in]
            n132 = Concatenate Strings(w219, w228, w227) -> (w220:string)
            n133 = local write "midVar_Content"(w220) -> ()
          }
          frame "body_e_Termiantion_TDD11" {
            n134 = local read "midVar_Content"() -> (w241:string)
            n135 = Concatenate Strings(w241, "        </ItemTest>\n") -> (w240:string)
            n136 = local write "midVar_Content"(w240) -> ()
          }
          frame "body_s_Cable area_TDD22" {
            n137 = local read "midVar_time"() -> (w247:string[])
            n138 = Index Array(array=w247, index #1=5 ("索引"), index #2=6 ("索引")) -> (element #1=w258:string, element #2=w255:string)
            n139 = Search and Replace String(input string="        <ItemTest ID=\"3\" name=\"Differential Impedance Cable（TDD22）\" startDateTime=\"@T1@\" endDateTime=\"@T2@\">\n            <TestResult BoardFlag=\"1\" ID=\"1\" SerialNumber=\"@L@\" ValueFlag=\"0\">\n                <Outcome value=\"@R@\"/>\n                <Description>NoDesc</Description>\n            </TestResult> \n", search string="@T1@" ("搜索字符串"), replace string=w258) -> (result string=w257:string)  [unwired: 5 in, 3 out]
            n140 = Search and Replace String(input string=w257, search string="@T2@" ("搜索字符串"), replace string=w255) -> (result string=w250:string)  [unwired: 5 in, 3 out]
            n141 = local read "input_str_label"() -> (w249:string)
            n142 = Search and Replace String(input string=w250, search string="@L@" ("搜索字符串"), replace string=w249) -> (result string=w245:string)  [unwired: 5 in, 3 out]
            n143 = local read "TDD"() -> (w242:string)
            n144 = Search and Replace String(input string=w245, search string="@R@" ("搜索字符串"), replace string=w242) -> (result string=w244:string)  [unwired: 5 in, 3 out]
            n145 = local read "midVar_Content"() -> (w254:string)
            n146 = Concatenate Strings(w254, w244) -> (w253:string)
            n147 = local write "midVar_Content"(w253) -> ()
          }
          frame "body_detail_Cable area_TDD22" {
            n148 = local read "input_path_dataSource"() -> (w273:path)
            n149 = local read "input_str_label"() -> (w276:string)
            n150 = local read "TDD"() -> (w262:string)
            n151 = local read "show_impspec"() -> (w264:string[])
            n152 = local read "midVar_Content"() -> (w283:string)
            n153 = Index Array(array=w264, index=1 ("索引")) -> (element=w261:string)
            n154 = Build Path(base path=w273, name or relative path="TXT" ("名称或相对路径")) -> (appended path=w272:path)
            n155 = Build Path(base path=w272, name or relative path="TDD22.txt" ("名称或相对路径")) -> (appended path=w269:path)
            n156 = Build Path(base path=w272, name or relative path="TDD11.txt" ("名称或相对路径")) -> (appended path=w268:path)
            n157 = case shown="假" "auto get refer point 2" {
              tunnel: w269 -> [_ w319]
              tunnel: w268 -> [_ w331]
              tunnel: ["cable points 2" w292] -> w265
              tunnel: ["terminal points 4" w293] -> w266
              frame False {
              }
              frame True {
                w288 = "\n"
                w296 = "point" ("delimiter (Tab)")
                w305 = "point" ("delimiter (Tab)")
                w328 = enum32{"Peaks", "Valleys"}."Valleys" ("peaks/valleys")
                w329 = 96.0 ("threshold")
                w330 = 15 ("PD width")
                n158 = local read "terminal points 4"() -> (w301:dbl[])
                n159 = local read "cable points 2"() -> (w302:dbl[])
                n160 = call-poly <vilib>:"Read From Spreadsheet File.vi"("file path (dialog if empty)"=w319) -> ("all rows"=w318:dbl[][])  [unwired: 6 in, 4 out]
                n161 = Index Array(array=w318, index (col)=0 ("禁用的索引 (列)")) -> (element=w314:dbl[])  [unwired: 1 in]
                n162 = call "terminal point.vi"("peaks/valleys"=w328, "threshold"=w329, "PD width"=w330, "TDD filePath"=w331) -> ("time low"=w323:dbl)  [unwired: 1 out]
                n163 = call "terminal point.vi"("peaks/valleys"=w328, "threshold"=w329, "PD width"=w330, "TDD filePath"=w319) -> ("time low"=w322:dbl)  [unwired: 1 out]
                n164 = Add(x=w323, y=w322) -> (x+y=w327:dbl)
                n165 = Number To Decimal String(number=w301) -> (decimal integer string=w303:string[])  [unwired: 1 in]
                n166 = Number To Decimal String(number=w302) -> (decimal integer string=w304:string[])  [unwired: 1 in]
                n167 = Divide(x=w327, y=2.0) -> (x/y=w320:dbl)
                n168 = Add(x=w320, y="width1 2") -> (x+y=w316:dbl)
                n169 = Add(x=w316, y="width2 2") -> (x+y=w315:dbl)
                n170 = Add(x=w315, y=2.0) -> (x+y=w313:dbl)
                n171 = call <userlib>:"1D Array to String__ogtk.vi"("delimiter (Tab)"=w305, "Array of Strings"=w303) -> ("delimited string"=w307:string)  [unwired: 9 in]
                n172 = Threshold 1D Array(2:w316, 3:w314) -> (0:w312:dbl)  [unwired: 1 in]
                n173 = Threshold 1D Array(2:w313, 3:w314) -> (0:w310:dbl)  [unwired: 1 in]
                n174 = Threshold 1D Array(2:w315, 3:w314) -> (0:w311:dbl)  [unwired: 1 in]
                n175 = call <userlib>:"1D Array to String__ogtk.vi"("delimiter (Tab)"=w305, "Array of Strings"=w304) -> ("delimited string"=w308:string)  [unwired: 9 in]
                n176 = Build Array(w312, w311) -> (w293:dbl[])
                n177 = Number To Decimal String(number=w293) -> (decimal integer string=w294:string[])  [unwired: 1 in]
                n178 = call <userlib>:"1D Array to String__ogtk.vi"("delimiter (Tab)"=w296, "Array of Strings"=w294) -> ("delimited string"=w298:string)  [unwired: 9 in]
                n179 = Build Array(w311, w310) -> (w292:dbl[])
                n180 = Number To Decimal String(number=w292) -> (decimal integer string=w295:string[])  [unwired: 1 in]
                n181 = call <userlib>:"1D Array to String__ogtk.vi"("delimiter (Tab)"=w296, "Array of Strings"=w295) -> ("delimited string"=w299:string)  [unwired: 9 in]
                n182 = Concatenate Strings("auto cable" ("字符串"), w299) -> (w290:string)
                n183 = Concatenate Strings("auto terminal:" ("字符串"), w298) -> (w291:string)
                n184 = Concatenate Strings("cable" ("字符串"), w308) -> (w287:string)
                n185 = Concatenate Strings("terminal:" ("字符串"), w307) -> (w289:string)
                n186 = Concatenate Strings(w291, w288, w290, w288, w289, w288, w287) -> ()  [unwired: 1 out]
              }
            }
            "terminal points 3" <- w266
            n187 = call "xmlFull.vi"("TDD?"=TRUE, "Points"=w265, "file path (dialog if empty)"=w268, "TDD spec"=w261, "SN"=w276, "数组"=string[] ["Cable area_TD:ZDD11", "Cable area_RD:ZDD11"], "second result"=w262) -> ("OutPutXml"=w281:string)  [unwired: 3 in]
            n188 = call "xmlFull.vi"("TDD?"=TRUE, "Points"=w265, "file path (dialog if empty)"=w269, "TDD spec"=w261, "SN"=w276, "数组"=string[] ["Cable area_TD:ZDD22", "Cable area_RD:ZDD22"], "second result"=w262) -> ("OutPutXml"=w274:string)  [unwired: 3 in]
            n189 = Concatenate Strings(w283, w281, w274) -> (w282:string)
            n190 = local write "midVar_Content"(w282) -> ()
          }
          frame "body_e_Cable area_TDD22" {
            n191 = local read "midVar_Content"() -> (w335:string)
            n192 = Concatenate Strings(w335, "        </ItemTest>\n") -> (w334:string)
            n193 = local write "midVar_Content"(w334) -> ()
          }
          frame "body_s_Termiantion_TDD22" {
            n194 = local read "midVar_time"() -> (w341:string[])
            n195 = Index Array(array=w341, index #1=4 ("索引"), index #2=5 ("索引")) -> (element #1=w352:string, element #2=w349:string)
            n196 = Search and Replace String(input string="        <ItemTest ID=\"4\" name=\"Differential Impedance Connector（TDD22）\" startDateTime=\"@T1@\" endDateTime=\"@T2@\">\n            <TestResult BoardFlag=\"1\" ID=\"1\" SerialNumber=\"@L@\" ValueFlag=\"0\">\n                <Outcome value=\"@R@\"/>\n                <Description>NoDesc</Description>\n            </TestResult> \n", search string="@T1@" ("搜索字符串"), replace string=w352) -> (result string=w351:string)  [unwired: 5 in, 3 out]
            n197 = Search and Replace String(input string=w351, search string="@T2@" ("搜索字符串"), replace string=w349) -> (result string=w344:string)  [unwired: 5 in, 3 out]
            n198 = local read "input_str_label"() -> (w343:string)
            n199 = Search and Replace String(input string=w344, search string="@L@" ("搜索字符串"), replace string=w343) -> (result string=w339:string)  [unwired: 5 in, 3 out]
            n200 = local read "TDD"() -> (w336:string)
            n201 = local read "midVar_Content"() -> (w348:string)
            n202 = Search and Replace String(input string=w339, search string="@R@" ("搜索字符串"), replace string=w336) -> (result string=w338:string)  [unwired: 5 in, 3 out]
            n203 = Concatenate Strings(w348, w338) -> (w347:string)
            n204 = local write "midVar_Content"(w347) -> ()
          }
          frame "body_detail_Termiantion_TDD22" {
            (unwired) string[] ["Termiantion_TD:ZDD11", "Termiantion_TD:ZDD22", "Termiantion_RD:ZDD11", "Termiantion_RD:ZDD22"]
            n205 = local read "input_path_dataSource"() -> (w365:path)
            n206 = Build Path(base path=w365, name or relative path="TXT" ("名称或相对路径")) -> (appended path=w372:path)
            n207 = local read "input_str_label"() -> (w362:string)
            n208 = local read "TDD"() -> (w358:string)
            n209 = Build Path(base path=w365, name or relative path="TXT" ("名称或相对路径")) -> (appended path=w376:path)
            n210 = local read "terminal points 2"() -> (w359:dbl[])
            n211 = Build Path(base path=w372, name or relative path="TDD22.txt" ("名称或相对路径")) -> (appended path=w370:path)
            n212 = local read "show_impspec"() -> (w357:string[])
            n213 = Build Path(base path=w376, name or relative path="TDD11.txt" ("名称或相对路径")) -> (appended path=w374:path)
            n214 = local read "midVar_Content"() -> (w360:string)
            n215 = Index Array(array=w357, index=0 ("索引")) -> (element=w355:string)
            n216 = call "xmlFull.vi"("TDD?"=TRUE, "Points"=w359, "file path (dialog if empty)"=w370, "TDD spec"=w355, "SN"=w362, "数组"=string[] ["Termiantion_TD:ZDD22", "Termiantion_RD:ZDD22"], "second result"=w358) -> ("OutPutXml"=w368:string)  [unwired: 3 in]
            n217 = call "xmlFull.vi"("TDD?"=TRUE, "Points"=w359, "file path (dialog if empty)"=w374, "TDD spec"=w355, "SN"=w362, "数组"=string[] ["Termiantion_TD:ZDD11", "Termiantion_RD:ZDD11"], "second result"=w358) -> ("OutPutXml"=w369:string)  [unwired: 3 in]
            n218 = Concatenate Strings(w360, w369, w368) -> (w361:string)
            n219 = local write "midVar_Content"(w361) -> ()
          }
          frame "body_e_Termiantion_TDD22" {
            n220 = local read "midVar_Content"() -> (w382:string)
            n221 = Concatenate Strings(w382, "        </ItemTest>\n") -> (w381:string)
            n222 = local write "midVar_Content"(w381) -> ()
          }
          frame "body_s_SDD21" {
            n223 = local read "midVar_time"() -> (w388:string[])
            n224 = Index Array(array=w388, index #1=0 ("索引"), index #2=1 ("索引")) -> (element #1=w399:string, element #2=w396:string)
            n225 = Search and Replace String(input string="        <ItemTest ID=\"5\" name=\"Differential Insertion Loss(SDD21)\" startDateTime=\"@T1@\" endDateTime=\"@T2@\">\n            <TestResult BoardFlag=\"1\" ID=\"1\" SerialNumber=\"@L@\" ValueFlag=\"0\">\n                <Outcome value=\"@R@\"/>\n                <Description>NoDesc</Description>\n            </TestResult>\n ", search string="@T1@" ("搜索字符串"), replace string=w399) -> (result string=w398:string)  [unwired: 5 in, 3 out]
            n226 = Search and Replace String(input string=w398, search string="@T2@" ("搜索字符串"), replace string=w396) -> (result string=w391:string)  [unwired: 5 in, 3 out]
            n227 = local read "input_str_label"() -> (w390:string)
            n228 = local read "SDD21"() -> (w383:string)
            n229 = Search and Replace String(input string=w391, search string="@L@" ("搜索字符串"), replace string=w390) -> (result string=w386:string)  [unwired: 5 in, 3 out]
            n230 = local read "midVar_Content"() -> (w395:string)
            n231 = Search and Replace String(input string=w386, search string="@R@" ("搜索字符串"), replace string=w383) -> (result string=w385:string)  [unwired: 5 in, 3 out]
            n232 = Concatenate Strings(w395, w385) -> (w394:string)
            n233 = local write "midVar_Content"(w394) -> ()
          }
          frame "body_detail_SDD21" {
            n234 = local read "input_path_dataSource"() -> (w412:path)
            n235 = local read "input_str_label"() -> (w411:string)
            n236 = Build Path(base path=w412, name or relative path="TXT" ("名称或相对路径")) -> (appended path=w416:path)
            n237 = local read "single spec"() -> (w405:T1)
            n238 = local read "SDD21"() -> (w406:string)
            n239 = Build Path(base path=w416, name or relative path="SDD21.txt" ("名称或相对路径")) -> (appended path=w414:path)
            n240 = local read "midVar_Content"() -> (w409:string)
            n241 = call "get single spec.vi"("single item name"="SDD21", "single spec"=w405) -> ("single spec"=w403:dbl[])  [unwired: 9 in]
            n242 = call "xmlFull.vi"("TDD?"=FALSE, "single spec"=w403, "file path (dialog if empty)"=w414, "limit type"=enum16{"上限", "下限"}."下限", "SN"=w411, "数组"=string[] ["Port1-Port2: TD-RD", "Port1-Port2: RD-TD"], "second result"=w406) -> ("OutPutXml"=w413:string)  [unwired: 3 in]
            n243 = Concatenate Strings(w409, w413) -> (w410:string)
            n244 = local write "midVar_Content"(w410) -> ()
          }
          frame "body_e_SDD21" {
            n245 = local read "midVar_Content"() -> (w422:string)
            n246 = Concatenate Strings(w422, "        </ItemTest>\n") -> (w421:string)
            n247 = local write "midVar_Content"(w421) -> ()
          }
          frame "body_s_SDD11" {
            n248 = local read "midVar_time"() -> (w428:string[])
            n249 = Index Array(array=w428, index #1=1 ("索引"), index #2=2 ("索引")) -> (element #1=w439:string, element #2=w436:string)
            n250 = Search and Replace String(input string="        <ItemTest ID=\"6\" name=\"Differential Return Loss(SDD11)\" startDateTime=\"@T1@\" endDateTime=\"@T2@\">\n            <TestResult BoardFlag=\"1\" ID=\"1\" SerialNumber=\"@L@\" ValueFlag=\"0\">\n                <Outcome value=\"@R@\"/>\n                <Description>NoDesc</Description>\n            </TestResult>\n ", search string="@T1@" ("搜索字符串"), replace string=w439) -> (result string=w438:string)  [unwired: 5 in, 3 out]
            n251 = Search and Replace String(input string=w438, search string="@T2@" ("搜索字符串"), replace string=w436) -> (result string=w431:string)  [unwired: 5 in, 3 out]
            n252 = local read "input_str_label"() -> (w430:string)
            n253 = local read "SDD11"() -> (w423:string)
            n254 = Search and Replace String(input string=w431, search string="@L@" ("搜索字符串"), replace string=w430) -> (result string=w426:string)  [unwired: 5 in, 3 out]
            n255 = local read "midVar_Content"() -> (w435:string)
            n256 = Search and Replace String(input string=w426, search string="@R@" ("搜索字符串"), replace string=w423) -> (result string=w425:string)  [unwired: 5 in, 3 out]
            n257 = Concatenate Strings(w435, w425) -> (w434:string)
            n258 = local write "midVar_Content"(w434) -> ()
          }
          frame "body_detail_SDD11" {
            n259 = local read "input_path_dataSource"() -> (w447:path)
            n260 = local read "input_str_label"() -> (w450:string)
            n261 = Build Path(base path=w447, name or relative path="TXT" ("名称或相对路径")) -> (appended path=w456:path)
            n262 = local read "single spec"() -> (w446:T1)
            n263 = local read "SDD11"() -> (w443:string)
            n264 = Build Path(base path=w456, name or relative path="SDD11.txt" ("名称或相对路径")) -> (appended path=w454:path)
            n265 = local read "midVar_Content"() -> (w449:string)
            n266 = call "get single spec.vi"("single item name"="SDD11", "single spec"=w446) -> ("single spec"=w444:dbl[])  [unwired: 9 in]
            n267 = call "xmlFull.vi"("TDD?"=FALSE, "single spec"=w444, "file path (dialog if empty)"=w454, "limit type"=enum16{"上限", "下限"}."上限", "SN"=w450, "数组"=string[] ["Port1-Port2: TD-RD", "Port1-Port2: RD-TD"], "second result"=w443) -> ("OutPutXml"=w453:string)  [unwired: 3 in]
            n268 = Concatenate Strings(w449, w453) -> (w448:string)
            n269 = local write "midVar_Content"(w448) -> ()
          }
          frame "body_e_SDD11" {
            n270 = local read "midVar_Content"() -> (w462:string)
            n271 = Concatenate Strings(w462, "        </ItemTest>\n") -> (w461:string)
            n272 = local write "midVar_Content"(w461) -> ()
          }
          frame "body_s_Next" {
            n273 = local read "midVar_time"() -> (w468:string[])
            n274 = Index Array(array=w468, index #1=6 ("索引"), index #2=7 ("索引")) -> (element #1=w479:string, element #2=w476:string)
            n275 = Search and Replace String(input string="        <ItemTest ID=\"7\" name=\"Multiple Disturber Near-end Crosstalk(Total NEXT)\" startDateTime=\"@T1@\" endDateTime=\"@T2@\">\n            <TestResult BoardFlag=\"1\" ID=\"1\" SerialNumber=\"@L@\" ValueFlag=\"0\">\n                <Outcome value=\"@R@\"/>\n                <Description>NoDesc</Description>\n            </TestResult>\n ", search string="@T1@" ("搜索字符串"), replace string=w479) -> (result string=w478:string)  [unwired: 5 in, 3 out]
            n276 = local read "NEXT"() -> (w466:string)
            n277 = Search and Replace String(input string=w478, search string="@T2@" ("搜索字符串"), replace string=w476) -> (result string=w471:string)  [unwired: 5 in, 3 out]
            n278 = local read "input_str_label"() -> (w470:string)
            n279 = Search and Replace String(input string=w471, search string="@L@" ("搜索字符串"), replace string=w470) -> (result string=w464:string)  [unwired: 5 in, 3 out]
            n280 = local read "midVar_Content"() -> (w475:string)
            n281 = Search and Replace String(input string=w464, search string="@R@" ("搜索字符串"), replace string=w466) -> (result string=w463:string)  [unwired: 5 in, 3 out]
            n282 = Concatenate Strings(w475, w463) -> (w474:string)
            n283 = local write "midVar_Content"(w474) -> ()
          }
          frame "body_detail_Next" {
            n284 = local read "input_path_dataSource"() -> (w494:path)
            n285 = local read "input_str_label"() -> (w492:string)
            n286 = Build Path(base path=w494, name or relative path="TXT" ("名称或相对路径")) -> (appended path=w496:path)
            n287 = local read "single spec"() -> (w485:T1)
            n288 = call "get single spec.vi"("single item name"="Next", "single spec"=w485) -> ("single spec"=w484:dbl[])  [unwired: 9 in]
            n289 = Build Path(base path=w496, name or relative path="NEXT.txt" ("名称或相对路径")) -> (appended path=w493:path)
            n290 = local read "NEXT"() -> (w483:string)
            n291 = call "xmlFull.vi"("TDD?"=FALSE, "single spec"=w484, "file path (dialog if empty)"=w493, "limit type"=enum16{"上限", "下限"}."上限", "SN"=w492, "数组"=string[] ["Next_TX-RX", "Next_RX-TX"], "second result"=w483) -> ("OutPutXml"=w490:string)  [unwired: 3 in]
            n292 = local read "midVar_Content"() -> (w489:string)
            n293 = Concatenate Strings(w489, w490) -> (w488:string)
            n294 = local write "midVar_Content"(w488) -> ()
          }
          frame "body_e_Next" {
            n295 = local read "midVar_Content"() -> (w502:string)
            n296 = Concatenate Strings(w502, "        </ItemTest>\n") -> (w501:string)
            n297 = local write "midVar_Content"(w501) -> ()
          }
          frame "body_s_SCD21" {
            n298 = local read "midVar_time"() -> (w508:string[])
            n299 = Index Array(array=w508, index #1=0 ("索引"), index #2=1 ("索引")) -> (element #1=w519:string, element #2=w516:string)
            n300 = Search and Replace String(input string="        <ItemTest ID=\"8\" name=\"Differential To Common-mode Conversion Loss(SCD21)\" startDateTime=\"@T1@\" endDateTime=\"@T2@\">\n            <TestResult BoardFlag=\"1\" ID=\"1\" SerialNumber=\"@L@\" ValueFlag=\"0\">\n                <Outcome value=\"@R@\"/>\n                <Description>NoDesc</Description>\n            </TestResult>\n ", search string="@T1@" ("搜索字符串"), replace string=w519) -> (result string=w518:string)  [unwired: 5 in, 3 out]
            n301 = Search and Replace String(input string=w518, search string="@T2@" ("搜索字符串"), replace string=w516) -> (result string=w511:string)  [unwired: 5 in, 3 out]
            n302 = local read "input_str_label"() -> (w510:string)
            n303 = local read "SDD21"() -> (w503:string)
            n304 = Search and Replace String(input string=w511, search string="@L@" ("搜索字符串"), replace string=w510) -> (result string=w506:string)  [unwired: 5 in, 3 out]
            n305 = local read "midVar_Content"() -> (w515:string)
            n306 = Search and Replace String(input string=w506, search string="@R@" ("搜索字符串"), replace string=w503) -> (result string=w505:string)  [unwired: 5 in, 3 out]
            n307 = Concatenate Strings(w515, w505) -> (w514:string)
            n308 = local write "midVar_Content"(w514) -> ()
          }
          frame "body_detail_SCD21" {
            n309 = local read "input_path_dataSource"() -> (w532:path)
            n310 = local read "input_str_label"() -> (w531:string)
            n311 = Build Path(base path=w532, name or relative path="TXT" ("名称或相对路径")) -> (appended path=w536:path)
            n312 = local read "single spec"() -> (w525:T1)
            n313 = local read "SDD21"() -> (w526:string)
            n314 = Build Path(base path=w536, name or relative path="SDD21.txt" ("名称或相对路径")) -> (appended path=w534:path)
            n315 = local read "midVar_Content"() -> (w529:string)
            n316 = call "get single spec.vi"("single item name"="SDD21", "single spec"=w525) -> ("single spec"=w523:dbl[])  [unwired: 9 in]
            n317 = call "xmlFull.vi"("TDD?"=FALSE, "single spec"=w523, "file path (dialog if empty)"=w534, "limit type"=enum16{"上限", "下限"}."下限", "SN"=w531, "数组"=string[] ["Port1-Port2: TD-RD", "Port1-Port2: RD-TD"], "second result"=w526) -> ("OutPutXml"=w533:string)  [unwired: 3 in]
            n318 = Concatenate Strings(w529, w533) -> (w530:string)
            n319 = local write "midVar_Content"(w530) -> ()
          }
          frame "body_e_SCD21" {
            n320 = local read "midVar_Content"() -> (w542:string)
            n321 = Concatenate Strings(w542, "        </ItemTest>\n") -> (w541:string)
            n322 = local write "midVar_Content"(w541) -> ()
          }
          frame "body_s_SCD21-SDD21" {
            n323 = local read "midVar_time"() -> (w548:string[])
            n324 = local read "input_str_label"() -> (w550:string)
            n325 = Index Array(array=w548, index #1=2 ("索引"), index #2=3 ("索引")) -> (element #1=w559:string, element #2=w556:string)
            n326 = Search and Replace String(input string="        <ItemTest ID=\"9\" name=\"Differential To Common-mode Conversion Loss-Differential Insertion Loss(SCD21-SDD21)\" startDateTime=\"@T1@\" endDateTime=\"@T2@\">\n            <TestResult BoardFlag=\"1\" ID=\"1\" SerialNumber=\"@L@\" ValueFlag=\"0\">\n                <Outcome value=\"@R@\"/>\n                <Description>NoDesc</Description>\n            </TestResult>\n ", search string="@T1@" ("搜索字符串"), replace string=w559) -> (result string=w558:string)  [unwired: 5 in, 3 out]
            n327 = Search and Replace String(input string=w558, search string="@T2@" ("搜索字符串"), replace string=w556) -> (result string=w551:string)  [unwired: 5 in, 3 out]
            n328 = Search and Replace String(input string=w551, search string="@L@" ("搜索字符串"), replace string=w550) -> (result string=w546:string)  [unwired: 5 in, 3 out]
            n329 = local read "SCD21-SDD21"() -> (w543:string)
            n330 = Search and Replace String(input string=w546, search string="@R@" ("搜索字符串"), replace string=w543) -> (result string=w545:string)  [unwired: 5 in, 3 out]
            n331 = local read "midVar_Content"() -> (w555:string)
            n332 = Concatenate Strings(w555, w545) -> (w554:string)
            n333 = local write "midVar_Content"(w554) -> ()
          }
          frame "body_detail_SCD21-SDD21" {
            n334 = local read "input_path_dataSource"() -> (w571:path)
            n335 = local read "SCD21-SDD21"() -> (w566:string)
            n336 = local read "input_str_label"() -> (w570:string)
            n337 = Build Path(base path=w571, name or relative path="TXT" ("名称或相对路径")) -> (appended path=w575:path)
            n338 = local read "single spec"() -> (w565:T1)
            n339 = Build Path(base path=w575, name or relative path="SCD21-SDD21.txt" ("名称或相对路径")) -> (appended path=w573:path)
            n340 = call "get single spec.vi"("single item name"="SCD21-SDD21", "single spec"=w565) -> ("single spec"=w563:dbl[])  [unwired: 9 in]
            n341 = call "xmlFull.vi"("single spec"=w563, "file path (dialog if empty)"=w573, "limit type"=enum16{"上限", "下限"}."上限", "SN"=w570, "数组"=string[] ["Port1-Port2: TD-RD", "Port1-Port2: RD-TD"], "second result"=w566) -> ("OutPutXml"=w572:string)  [unwired: 4 in]
            n342 = local read "midVar_Content"() -> (w568:string)
            n343 = Concatenate Strings(w568, w572) -> (w567:string)
            n344 = local write "midVar_Content"(w567) -> ()
          }
          frame "body_e_SCD21-SDD21" {
            n345 = local read "midVar_Content"() -> (w581:string)
            n346 = Concatenate Strings(w581, "        </ItemTest>\n") -> (w580:string)
            n347 = local write "midVar_Content"(w580) -> ()
          }
          frame "tail" {
            # "</ResultSet>\n    <TestProgram Productline=\"XT-113\" Product=\"SFP+\">\n        <c:Definition name=\"HPTS\" version=\"6.0\">\n            <c:Description>NoDesc</c:Description> \n        </c:Definition>\n    </TestProgram>\n    <!--  ATE--> \n    <TestStation AteName=\"TDR\" AteVersion=\"1.001\" /> \n    <!--  SerialNumber--> \n    <UUT UutType=\"hardware\">\n        <SerialNumber>@L@</SerialNumber> \n        <ItemName>SFP+</ItemName>\n        <ItemCode>@C@</ItemCode> \n    </UUT>\n    <WorkOrder>\n        <WorkItem name=\"a\">\n            <c:Datum xsi:type=\"c:string\">\n                <c:Value>SPZS06311C1</c:Value> \n            </c:Datum>\n        </WorkItem>\n    </WorkOrder>\n</TestResults"
            n348 = Concatenate Strings("\"" ("字符串"), "FileVer", "\"" ("字符串")) -> (w586:string)
            n349 = local read "input_str_product"() -> (w608:string)
            n350 = Search and Replace String(input string="    </ResultSet>\n    <TestProgram Productline=\"XT-113\" Product=\"SFP+\">\n        <c:Definition name=\"VNA\" version=@Ver@>\n            <c:Description>@Path@</c:Description> \n        </c:Definition>\n    </TestProgram>\n    <!--  ATE--> \n    <TestStation AteName=@PCName@ AteVersion=\"1.001\" /> \n    <!--  SerialNumber--> \n    <UUT UutType=\"hardware\">\n        <SerialNumber>@L@</SerialNumber> \n        <ItemName>SFP+</ItemName>\n        <ItemCode>@C@</ItemCode> \n    </UUT>\n    <WorkOrder>\n        <WorkItem name=\"a\">\n            <c:Datum xsi:type=\"c:string\">\n                <c:Value>SPZS06311C1</c:Value> \n            </c:Datum>\n        </WorkItem>\n    </WorkOrder>\n</TestResults>", search string="@Ver@" ("搜索字符串"), replace string=w586) -> (result string=w595:string)  [unwired: 5 in, 3 out]
            n351 = call "PCsName.vi"() -> ("Computer Name"=w585:string)
            n352 = Search and Replace String(input string=w595, search string="@Path@" ("搜索字符串"), replace string="FilePath") -> (result string=w593:string)  [unwired: 5 in, 3 out]
            n353 = local read "input_str_label"() -> (w605:string)
            n354 = Concatenate Strings("\"" ("字符串"), w585, "\"" ("字符串")) -> (w582:string)
            n355 = Search and Replace String(input string=w593, search string="@PCName@" ("搜索字符串"), replace string=w582) -> (result string=w591:string)  [unwired: 5 in, 3 out]
            n356 = Search and Replace String(input string=w591, search string="@P@" ("搜索字符串"), replace string=w608) -> (result string=w607:string)  [unwired: 5 in, 3 out]
            n357 = Search and Replace String(input string=w607, search string="@L@" ("搜索字符串"), replace string=w605) -> (result string=w600:string)  [unwired: 5 in, 3 out]
            n358 = local read "input_str_CustomerPN"() -> (w598:string)
            n359 = local read "midVar_Content"() -> (w604:string)
            n360 = Search and Replace String(input string=w600, search string="@C@" ("搜索字符串"), replace string=w598) -> (result string=w601:string)  [unwired: 5 in, 3 out]
            n361 = Concatenate Strings(w604, w601) -> (w603:string)
            n362 = local write "midVar_Content"(w603) -> ()
          }
          frame "end" {
            n363 = local read "midVar_Content"() -> (w611:string)
            n364 = Open/Create/Replace File(file path (use dialog)="路径", operation (0:open)=T2."open or create" ("操作(0:open)")) -> (refnum out=w615:refnum<file>)  [unwired: 4 in, 2 out]
            n365 = Text to UTF-8(11:w611) -> (3:w610:string)  [unwired: 1 in, 1 out]
            n366 = Write to Text File(file (use dialog)=w615, text=w610) -> (refnum out=w614:refnum<file>)  [unwired: 2 in, 2 out]
            n367 = Close File(refnum=w614) -> ()  [unwired: 1 in, 2 out]
          }
        }
        n368 = local write "midVar_state"(w68) -> ()
      }
    }
  }
